vi "LeCroy.Configure Channel.vi"(4 "Enable":bool=TRUE, 5 "Channel":u16(ring) items=["Channel 1", "Channel 2", "Channel 3", "Channel 4"], 6 "Coupling":u16(ring) items=["A1M", "D1M", "D50", "Ground", "DC", "AC"], 7 "Bandwidth":u16(ring) items=["Full", "20MHZ", "25MHZ", "200MHZ", "250MHZ", "1GHZ", "3GHZ", "4GHZ"], 8 "Error In":errorcluster, 10 "Vertical Range":dbl=10.0, 11 "LeCroy.Session in":T1) -> (0 "Error Out":errorcluster, 3 "LeCroy.Session out":T1)   [LabVIEW 2018]
uses:
  typedefs/LeCroy.Session.ctl
  <instrlib>/LeCroy Wave Series/LeCroy Wave Series.lvlib
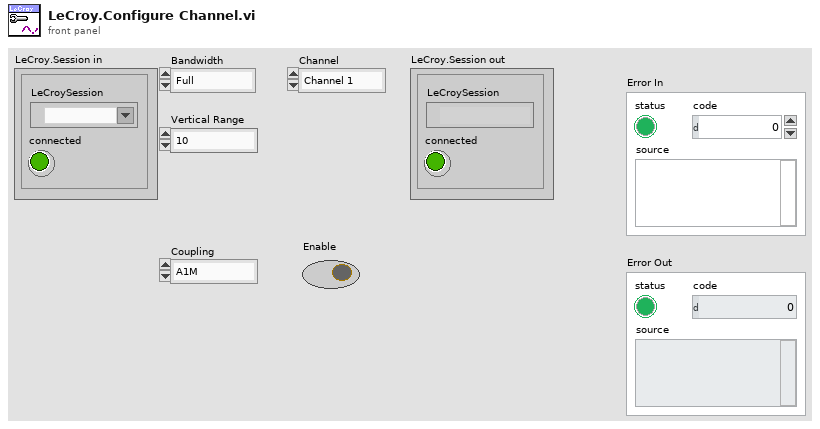
[diagram p1: front panel]
types:
  T1 = typedef "LeCroy.Session.ctl" = cluster{"LeCroySession":refnum<visa-resource-name>, "connected":bool}
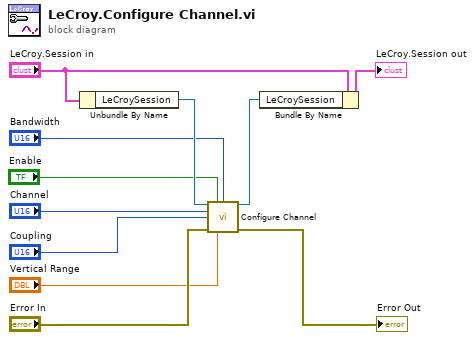
[diagram p0: block diagram]
diagram:
  n1 = Unbundle By Name("LeCroy.Session in") -> ("LeCroySession"=w9:refnum<visa-resource-name>)
  n2 = call <instrlib>:"Configure Channel.vi"("VISA resource name"=w9, "Enable Channel (T:On)"="Enable", "Bandwidth (0: Full)"="Bandwidth", "Channel (0: Channel 1)"="Channel", "Vertical Coupling (0: A1M)"="Coupling", "error in (no error)"="Error In", "Vertical Range (10.0 V)"="Vertical Range") -> ("VISA resource name out"=w8:refnum<visa-resource-name>, "error out"=→"Error Out":errorcluster)  [unwired: 7 in]
  n3 = Bundle By Name(cluster="LeCroy.Session in", "LeCroySession"=w8) -> (→"LeCroy.Session out":T1)
